vi "showStimulus.vi"(8 "error in (no error)":errorcluster, 11 "Stimulus in":refnum<class "Stimulus.lvclass">) -> (0 "error out":errorcluster, 3 "Stimulus out":refnum<class "Stimulus.lvclass">)   [LabVIEW 2014, in "Stimulus.lvclass"]
uses:
  Stimulus.lvclass
  Stimulus.lvclass/Stimulus.ctl
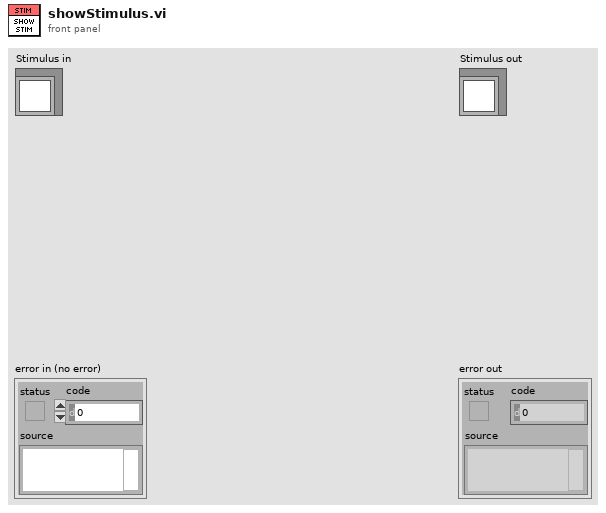
[diagram p1: front panel]
types:
  T1 = typedef "IMAQ Image.ctl" = refnum<image>
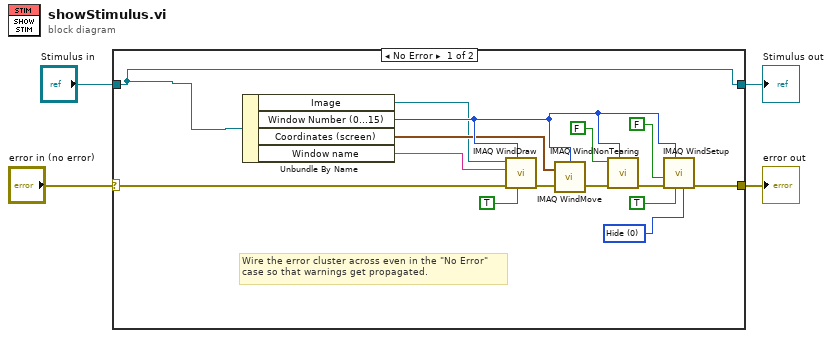
[diagram p0: block diagram]
diagram:
  n1 = case shown="No Error" "error in (no error)" {
    selector: "error in (no error)" -> [w19 w21]
    tunnel: [w18 w21] -> w3
    tunnel: [w5 w20] -> w1
    tunnel: "Stimulus in" -> [w5 w20]
    frame No Error {
      w11 = 0 items=["Hide", "Show", "No change"] ("Scrollbars (No change)")
      # "Wire the error cluster across even in the \"No Error\"\ncase so that warnings get propagated."
      n2 = Unbundle By Name(w5) -> ("Image"=w7:T1, "Window Number (0...15)"=w9:i32, "Coordinates (screen)"=w8:cluster{"X Position":i32, "Y Position":i32}, "Window name"=w6:string)
      n3 = call "IMAQ WindDraw"("Resize to Image Size? (Y)"=TRUE, "Window Number (0...15)"=w9, "error in (no error)"=w19, "Title"=w6, "Image"=w7) -> ("error out"=w16:errorcluster)  [unwired: 5 in, 1 out]
      n4 = call "IMAQ WindMove"("Window Number (0...15)"=w9, "Coordinates (screen)"=w8, "error in (no error)"=w16) -> ("error out"=w15:errorcluster)  [unwired: 2 in, 1 out]
      n5 = call "IMAQ WindNonTearing"("Window Number"=w9, "error in (no error)"=w15, "NonTearing? (True)"=FALSE) -> ("error out"=w10:errorcluster)  [unwired: 7 in, 1 out]
      n6 = call "IMAQ WindSetup"("Scrollbars (No change)"=w11, "Window is floating? (No)"=TRUE, "Window Number (0...15)"=w9, "error in (no error)"=w10, "Window has title bar? (Yes)"=FALSE) -> ("error out"=w18:errorcluster)  [unwired: 6 in]
    }
    frame Error {
    }
  }
  "error out" <- w3
  "Stimulus out" <- w1
